vi "Remove XLSX Empty Rows.vi"(8 "error in (no error)":errorcluster, 11 "Array in":string[][](array[string])) -> (0 "error out":errorcluster, 1 "Removed Row Indices":i32[](array[numeric]), 3 "Array out":string[][](array[string]))   [LabVIEW 2021, in "Files.lvlib"]
doc: "Fills table with copies of the single-copy value of multicell-spanning super-cell."
uses:
  Files.lvlib
panel:
  # "see the AlliGator License on the block diagram (Ctrl+E or Window:Show Block Diagram)"
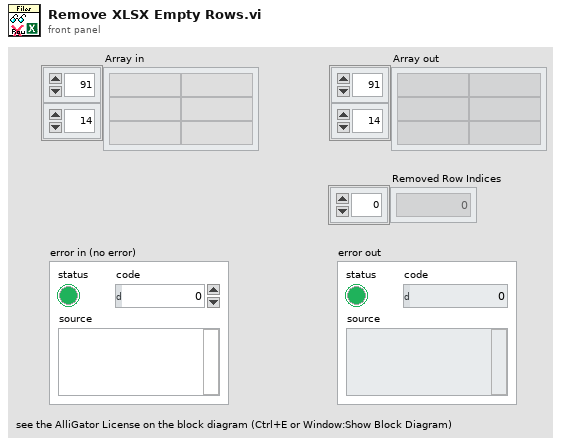
[diagram p1: front panel]
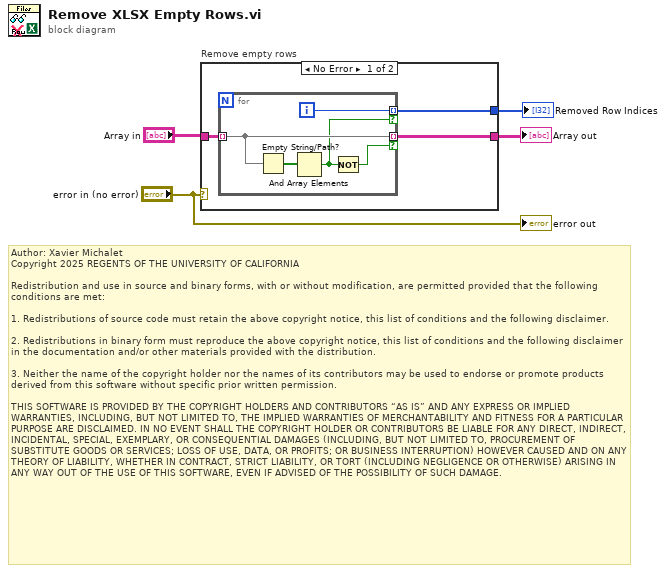
[diagram p0: block diagram]
diagram:
  # "Author: Xavier Michalet\nCopyright 2025 REGENTS OF THE UNIVERSITY OF CALIFORNIA\n\nRedistribution and use in source and binary forms, with or without modification, are permitted provided that the following conditions are met:\n\n1. Redistributions of source code must retain the above copyright notice, this list of conditions and the following disclaimer.\n\n2. Redistributions in binary form must reproduce the above copyright notice, this list of conditions and the following disclaimer in the documentation and/or other materials provided with the distribution.\n\n3. Neither the name of the copyright holder nor the names of its contributors may be used to endorse or promote products derived from this software without specific prior written permission.\n\nTHIS SOFTWARE IS PROVIDED BY THE COPYRIGHT HOLDERS AND CONTRIBUTORS “AS IS” AND ANY EXPRESS OR IMPLIED WARRANTIES, INCLUDING, BUT NOT LIMITED TO, THE IMPLIED WARRANTIES OF MERCHANTABILITY AND FITNESS FOR A PARTICULAR PURPOSE ARE DISCLAIMED. IN NO EVENT SHALL THE COPYRIGHT HOLDER OR CONTRIBUTORS BE LIABLE FOR ANY DIRECT, INDIRECT, INCIDENTAL, SPECIAL, EXEMPLARY, OR CONSEQUENTIAL DAMAGES (INCLUDING, BUT NOT LIMITED TO, PROCUREMENT OF SUBSTITUTE GOODS OR SERVICES; LOSS OF USE, DATA, OR PROFITS; OR BUSINESS INTERRUPTION) HOWEVER CAUSED AND ON ANY THEORY OF LIABILITY, WHETHER IN CONTRACT, STRICT LIABILITY, OR TORT (INCLUDING NEGLIGENCE OR OTHERWISE) ARISING IN ANY WAY OUT OF THE USE OF THIS SOFTWARE, EVEN IF ADVISED OF THE POSSIBILITY OF SUCH DAMAGE."
  n1 = case "Remove empty rows" shown="No Error" "error in (no error)" {
    tunnel: "Array in" -> [w7 w13]
    tunnel: [w5 w13] -> w2
    tunnel: [w6 _] -> w1
    frame No Error {
      n2 = for {
        tunnel: w7 -> [w11] mode=indexing
        tunnel: [w11] -> w5 mode=indexing if=w9
        tunnel: [w10] -> w6 mode=indexing if=w8
        i -> [w10]
        n3 = Empty String/Path?(string/path=w11) -> (empty?=w12:bool[])
        n4 = And Array Elements(Boolean array=w12) -> (logical AND=w8:bool)
        n5 = Not(x=w8) -> (.not. x?=w9:bool)
      }
    }
    frame Error {
    }
  }
  "Array out" <- w2
  "Removed Row Indices" <- w1
  "error out" <- "error in (no error)"
